vi "Begin.vi"(11 "Image Size":T1=enum."320x240") -> (0 "error out":errorcluster)   [LabVIEW 2012]
doc: "Called before other user functions, this VI is expected to open initial I/O refnums, load in file data, and do all program initialization. Notice that the <B>error out</B> terminal is simply used for data flow. Wiring it to other structures or subVIs ensures that this VI runs first."
uses:
  <vilib>/Rock Robotics/WPI/Camera/WPI_CameraImageSize.ctl
  <vilib>/Rock Robotics/WPI/DriverStation/WPI_DriverStationRobotMode2.ctl
  <vilib>/Rock Robotics/SystemInterfaces/DIO/FPGA_DIOPWMChannel.ctl
  <vilib>/Rock Robotics/WPI/Joystick/WPI_JoystickDeviceEnum.ctl
  <vilib>/Rock Robotics/WPI/Relay/WPI_RelayDirection.ctl
  <vilib>/Rock Robotics/SystemInterfaces/DIO/FPGA_DIORelayChannel.ctl
  <vilib>/Rock Robotics/SystemInterfaces/Typedef/FPGA_TypedefDigitalModule.ctl
  <vilib>/Rock Robotics/SystemInterfaces/AI/FPGA_AIChannel.ctl
  <vilib>/Rock Robotics/SystemInterfaces/AI/FPGA_AIGyroChannel.ctl
  <vilib>/Rock Robotics/SystemInterfaces/DIO/FPGA_DIOChannel.ctl
  Robot Global Data.vi
  <vilib>/Rock Robotics/WPI/MotorControl/WPI_MotorControlOpen Victor.vi
  <vilib>/Rock Robotics/WPI/Camera/WPI_CameraFrameRate.ctl
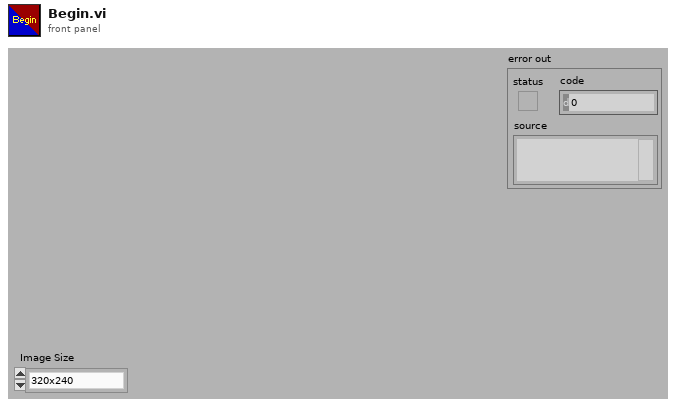
[diagram p1: front panel]
types:
  T1 = typedef "WPI_CameraImageSize.ctl" = enum16{"640x480", "320x240", "160x120"}
  T2 = typedef "FPGA_TypedefDigitalModule.ctl" = enum16{"Digital Module 1", "Digital Module 2"}
  T3 = typedef "FPGA_DIOPWMChannel.ctl" = enum8{"PWM 1", "PWM 2", "PWM 3", "PWM 4", "PWM 5", "PWM 6", "PWM 7", "PWM 8", "PWM 9", "PWM 10", "Invalid"}
  T4 = typedef "FPGA_DIORelayChannel.ctl" = enum8{"Relay 1", "Relay 2", "Relay 3", "Relay 4", "Relay 5", "Relay 6", "Relay 7", "Relay 8", "Invalid"}
  T5 = typedef "WPI_RelayDirection.ctl" = enum16{"Both directions", "Forward only", "Reverse only"}
  T6 = typedef "FPGA_DIOChannel.ctl" = enum8{"DIO 1", "DIO 2", "DIO 3", "DIO 4", "DIO 5", "DIO 6", "DIO 7", "DIO 8", "DIO 9", "DIO 10", "DIO 11", "DIO 12", "DIO 13", "DIO 14", "Invalid"}
  T7 = typedef "FPGA_AIChannel.ctl" = enum8{"AI 1", "AI 2", "AI 3", "AI 4", "AI 5", "AI 6", "AI 7", "AI 8", "Invalid"}
  T8 = typedef "FPGA_AIGyroChannel.ctl" = enum8{"AI 1", "AI 2", "Invalid"}
  T9 = typedef "WPI_JoystickDeviceEnum.ctl" = enum16{"USB 1", "USB 2", "USB 3", "USB 4", "Kinect 1", "Kinect 2"}
  T10 = typedef "WPI_DriverStationRobotMode2.ctl" = enum16{"Autonomous Disabled", "Autonomous Enabled", "Teleop Disabled", "Teleop Enabled", "Timeout", "Finish", "Test Disabled", "Test Enabled"}
  T11 = typedef "WPI_RelayDevRef.ctl" = cluster{"DevStatus":errorcluster, "Relay Channel":T4, "Digital Module":T2, "Relay Direction":T5}
  T12 = typedef "WPI_CameraFrameRate.ctl" = u32
  T13 = typedef "WPI_CameraDevRef.ctl" = cluster{"Camera Address":string, "CameraStatus":errorcluster, "Acquire Image Notifier":refnum<notifier>}
  T14 = typedef "WPI_MotorControlDeviceRef.ctl" = cluster{"DeviceStatus":errorcluster, "Type":enum16{"PWM", "CAN"}, "PWM":cluster{"Digital Module":T2, "PWM Channel":T3, "DeadBand":T15}, "CAN":cluster{"Device Number":u8, "Control Mode":T16, "Semaphore":T17, "Max Vout":dbl}, "Invert":bool, "TransformRef":T18, "InvTransformRef":T18}
  T15 = typedef "WPI_PWMDeadband.ctl" = cluster{"Name":string, "maxPositivePwm":i32, "minPositivePwm":i32, "centerPwm":i32, "maxNegativePwm":i32, "minNegativePwm":i32, "angularRange":u16}
  T16 = typedef "WPI_CANJaguar_ControlMode.ctl" = enum8{"Percent VBus", "Current", "Speed", "Position", "Voltage"}
  T17 = typedef "Semaphore RefNum" = refnum<k1>
  T18 = typedef "WPI_PWMTransform_ConPane.ctl" = refnum<vi>
  T19 = cluster{"Setpoint 1":dbl, "Setpoint 2":dbl, "Setpoint 3":dbl, "Setpoint 4":dbl, "RotLow":dbl, "RotHigh":dbl, "ExtLow":dbl, "ExtHigh":dbl}
  T20 = cluster{"FlipperLeftUp":dbl, "FlipperLeftDown":dbl, "FlipperRightUp":dbl, "FlipperRightDown":dbl, "KickerLeftBack":dbl, "KickerLeftForward":dbl, "KickerRightBack":dbl, "KickerRightForward":dbl}
  T21 = typedef "WPI_JoystickDevRef.ctl" = cluster{"Device":T9}
  T22 = typedef "WPI_ServoDeviceRef.ctl" = cluster{"DeviceStatus":errorcluster, "Digital Module":T2, "PWM Channel":T3, "DeadBand":T15}
  T23 = typedef "WPI_DigitalInputDevRef.ctl" = cluster{"DevStatus":errorcluster, "DIO Channel":T6, "Digital Module":T2}
  T24 = typedef "WPI_AnalogChannelDevRef.ctl" = cluster{"DevStatus":errorcluster, "Analog Module":T25, "Analog Channel":T7}
  T25 = typedef "FPGA_TypedefAnalogModule.ctl" = enum16{"Analog Module 1", "Analog Module 2"}
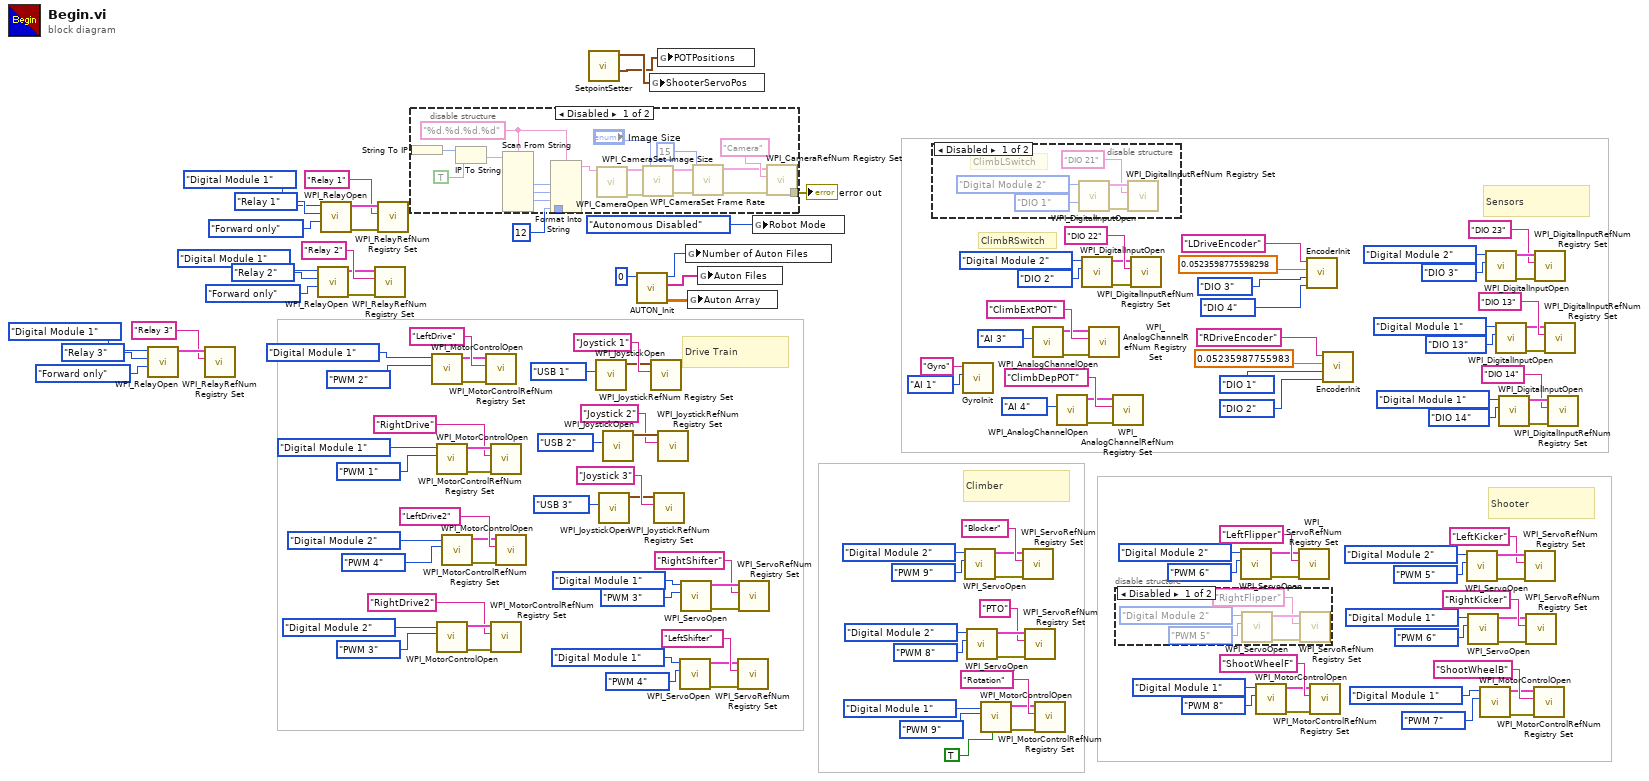
[diagram p0: block diagram]
diagram:
  # "ClimbRSwitch"
  # "Shooter"
  # "Drive Train"
  # "Climber"
  # "Sensors"
  n1 = call <vilib>:"WPI_RelayOpen.vi"("Relay Direction"=WPI_RelayDirection."Forward only", "Relay Channel"=FPGA_DIORelayChannel."Relay 3", "Digital Module (Module 1)"=FPGA_TypedefDigitalModule."Digital Module 1") -> ("RelayDevRef"=w14:T11)  [unwired: 7 in, 1 out]
  n2 = call <vilib>:"WPI_RelayRefNum Registry Set.vi"("refnum name"="Relay 3", "RelayDevRef"=w14) -> ()  [unwired: 8 in, 2 out]
  n3 = call <vilib>:"WPI_RelayOpen.vi"("Relay Direction"=WPI_RelayDirection."Forward only", "Relay Channel"=FPGA_DIORelayChannel."Relay 2", "Digital Module (Module 1)"=FPGA_TypedefDigitalModule."Digital Module 1") -> ("error out"=w106:errorcluster, "RelayDevRef"=w107:T11)  [unwired: 7 in]
  n4 = call <vilib>:"WPI_RelayOpen.vi"("Relay Direction"=WPI_RelayDirection."Forward only", "Relay Channel"=FPGA_DIORelayChannel."Relay 1", "Digital Module (Module 1)"=FPGA_TypedefDigitalModule."Digital Module 1") -> ("error out"=w64:errorcluster, "RelayDevRef"=w63:T11)  [unwired: 7 in]
  n5 = call <vilib>:"WPI_RelayRefNum Registry Set.vi"("error in (no error)"=w106, "refnum name"="Relay 2", "RelayDevRef"=w107) -> ()  [unwired: 7 in, 2 out]
  n6 = call <vilib>:"WPI_RelayRefNum Registry Set.vi"("error in (no error)"=w64, "refnum name"="Relay 1", "RelayDevRef"=w63) -> ()  [unwired: 7 in, 2 out]
  n7 = disable-structure shown="Disabled" {
    disable-tunnel: 12 ("Compression") -> [w155 _]
    disable-tunnel: [w145 _] -> w65
    frame Disabled {
      w154 = "%d.%d.%d.%d" ("format string")
      n8 = String To IP() -> (0:w161:u32)  [unwired: 1 in]
      n9 = IP To String(1:TRUE ("dot notation? (F)"), 2:w161) -> (0:w159:string)
      n10 = Scan From String(format string=w154, input string=w159) -> (output 1=w158:i32, output 2=w157:i32, output 3=w156:i32)  [unwired: 7 in, 3 out]
      n11 = Format Into String(format string=w154, w158, w157, w156, w155) -> (resulting string=w153:string)  [unwired: 2 in, 1 out]
      n12 = call <vilib>:"WPI_CameraOpen.vi"("Camera Address"=w153) -> ("error out"=w152:errorcluster, "CameraDevRef"=w151:T13)  [unwired: 1 in, 8 out]
      n13 = call <vilib>:"WPI_CameraSet Image Size.vi"("error in (no error)"=w152, "Image Size"="Image Size", "CameraDevRef"=w151) -> ("error out"=w149:errorcluster, "CameraDevRef Out"=w150:T13)  [unwired: 7 out]
      n14 = call <vilib>:"WPI_CameraSet Frame Rate.vi"("error in (no error)"=w149, "Frame Rate (fps)"=T12 15, "CameraDevRef"=w150) -> ("error out"=w148:errorcluster, "CameraDevRef Out"=w147:T13)  [unwired: 7 out]
      n15 = call <vilib>:"WPI_CameraRefNum Registry Set.vi"("error in (no error)"=w148, "refnum name"="Camera", "CameraDevRef"=w147) -> ("error out"=w145:errorcluster)  [unwired: 8 out]
    }
    frame Enabled {
    }
  }
  "error out" <- w65
  n16 = call-poly <vilib>:"WPI_MotorControlOpen.vi"("PWM Channel"=FPGA_DIOPWMChannel."PWM 2", "Digital Module (Module 1)"=FPGA_TypedefDigitalModule."Digital Module 1") -> ("error out"=w132:errorcluster, "MotorControlDeviceRef"=w133:T14)  [unwired: 8 in]
  n17 = call-poly <vilib>:"WPI_MotorControlOpen.vi"("PWM Channel"=FPGA_DIOPWMChannel."PWM 1", "Digital Module (Module 1)"=FPGA_TypedefDigitalModule."Digital Module 1") -> ("error out"=w139:errorcluster, "MotorControlDeviceRef"=w138:T14)  [unwired: 8 in]
  n18 = call-poly <vilib>:"WPI_MotorControlOpen.vi"("PWM Channel"=FPGA_DIOPWMChannel."PWM 3", "Digital Module (Module 1)"=FPGA_TypedefDigitalModule."Digital Module 2") -> ("error out"=w121:errorcluster, "MotorControlDeviceRef"=w120:T14)  [unwired: 8 in]
  n19 = call-poly <vilib>:"WPI_MotorControlOpen.vi"("PWM Channel"=FPGA_DIOPWMChannel."PWM 4", "Digital Module (Module 1)"=FPGA_TypedefDigitalModule."Digital Module 2") -> ("error out"=w112:errorcluster, "MotorControlDeviceRef"=w113:T14)  [unwired: 8 in]
  n20 = call <vilib>:"WPI_MotorControlRefNum Registry Set.vi"("error in (no error)"=w132, "refnum name"="LeftDrive", "MotorControlDevRef"=w133) -> ()  [unwired: 7 in, 2 out]
  n21 = call <vilib>:"WPI_MotorControlRefNum Registry Set.vi"("error in (no error)"=w139, "refnum name"="RightDrive", "MotorControlDevRef"=w138) -> ()  [unwired: 7 in, 2 out]
  n22 = call <vilib>:"WPI_MotorControlRefNum Registry Set.vi"("error in (no error)"=w121, "refnum name"="RightDrive2", "MotorControlDevRef"=w120) -> ()  [unwired: 7 in, 2 out]
  n23 = call <vilib>:"WPI_MotorControlRefNum Registry Set.vi"("error in (no error)"=w112, "refnum name"="LeftDrive2", "MotorControlDevRef"=w113) -> ()  [unwired: 7 in, 2 out]
  n24 = call "SetpointSetter.vi"() -> ("Arm Pos"=w1:T19, "Shooter Servo Pos"=w2:T20)  [unwired: 10 in]
  n25 = call <vilib>:"WPI_JoystickOpen.vi"("JoystickDevice"=WPI_JoystickDeviceEnum."USB 1") -> ("JoystickDevRef"=w123:T21)  [unwired: 10 in]
  n26 = call <vilib>:"WPI_JoystickOpen.vi"("JoystickDevice"=WPI_JoystickDeviceEnum."USB 3") -> ("JoystickDevRef"=w129:T21)  [unwired: 10 in]
  n27 = call <vilib>:"WPI_JoystickOpen.vi"("JoystickDevice"=WPI_JoystickDeviceEnum."USB 2") -> ("JoystickDevRef"=w128:T21)  [unwired: 10 in]
  n28 = call "AUTON_Init.vi"("Default File"=0) -> ("Auton Array"=w140:dbl[][], "Auton Files"=w141:string[], "Number of Auton Files"=w142:i64)  [unwired: 8 in]
  n29 = global write "Robot Global Data.vi" "ShooterServoPos"(w2) -> ()
  n30 = call <vilib>:"WPI_JoystickRefNum Registry Set.vi"("refnum name"="Joystick 1", "JoystickDevRef"=w123) -> ()  [unwired: 8 in, 2 out]
  n31 = call <vilib>:"WPI_JoystickRefNum Registry Set.vi"("refnum name"="Joystick 3", "JoystickDevRef"=w129) -> ()  [unwired: 8 in, 2 out]
  n32 = global write "Robot Global Data.vi" "POTPositions"(w1) -> ()
  n33 = call <vilib>:"WPI_JoystickRefNum Registry Set.vi"("refnum name"="Joystick 2", "JoystickDevRef"=w128) -> ()  [unwired: 8 in, 2 out]
  n34 = call <vilib>:"WPI_ServoOpen.vi"("PWM Channel"=FPGA_DIOPWMChannel."PWM 4", "Digital Module (Module 1)"=FPGA_TypedefDigitalModule."Digital Module 1") -> ("error out"=w105:errorcluster, "ServoDeviceRef"=w98:T22)  [unwired: 8 in]
  n35 = call <vilib>:"WPI_ServoOpen.vi"("PWM Channel"=FPGA_DIOPWMChannel."PWM 3", "Digital Module (Module 1)"=FPGA_TypedefDigitalModule."Digital Module 1") -> ("error out"=w104:errorcluster, "ServoDeviceRef"=w103:T22)  [unwired: 8 in]
  n36 = global write "Robot Global Data.vi" "Number of Auton Files"(w142) -> ()
  n37 = global write "Robot Global Data.vi" "Auton Array"(w140) -> ()
  n38 = global write "Robot Global Data.vi" "Auton Files"(w141) -> ()
  n39 = call <vilib>:"WPI_ServoRefNum Registry Set.vi"("error in (no error)"=w105, "refnum name"="LeftShifter", "ServoDeviceRef"=w98) -> ()  [unwired: 7 in, 2 out]
  n40 = call <vilib>:"WPI_ServoRefNum Registry Set.vi"("error in (no error)"=w104, "refnum name"="RightShifter", "ServoDeviceRef"=w103) -> ()  [unwired: 7 in, 2 out]
  n41 = global write "Robot Global Data.vi" "Robot Mode"(WPI_DriverStationRobotMode2."Autonomous Disabled" ("Robot Mode")) -> ()
  n42 = disable-structure shown="Disabled" {
    frame Disabled {
      # "ClimbLSwitch"
      n43 = call <vilib>:"WPI_DigitalInputOpen.vi"("DIO Channel"=FPGA_DIOChannel."DIO 1", "Digital Module (Module 1)"=FPGA_TypedefDigitalModule."Digital Module 2") -> ("error out"=w165:errorcluster, "DigitalInputDevRef"=w166:T23)  [unwired: 8 in]
      n44 = call <vilib>:"WPI_DigitalInputRefNum Registry Set.vi"("error in (no error)"=w165, "refnum name"="DIO 21", "DigitalInputDevRef"=w166) -> ()  [unwired: 7 in, 2 out]
    }
    frame Enabled {
    }
  }
  n45 = call "GyroInit.vi"("refnum name"="Gyro", "Analog Channel"=FPGA_AIGyroChannel."AI 1") -> ()  [unwired: 8 in]
  n46 = call <vilib>:"WPI_ServoOpen.vi"("PWM Channel"=FPGA_DIOPWMChannel."PWM 9", "Digital Module (Module 1)"=FPGA_TypedefDigitalModule."Digital Module 2") -> ("error out"=w4:errorcluster, "ServoDeviceRef"=w5:T22)  [unwired: 8 in]
  n47 = call <vilib>:"WPI_ServoOpen.vi"("PWM Channel"=FPGA_DIOPWMChannel."PWM 8", "Digital Module (Module 1)"=FPGA_TypedefDigitalModule."Digital Module 2") -> ("error out"=w83:errorcluster, "ServoDeviceRef"=w82:T22)  [unwired: 8 in]
  n48 = call-poly <vilib>:"WPI_MotorControlOpen.vi"("Invert"=TRUE, "PWM Channel"=FPGA_DIOPWMChannel."PWM 9", "Digital Module (Module 1)"=FPGA_TypedefDigitalModule."Digital Module 1") -> ("error out"=w88:errorcluster, "MotorControlDeviceRef"=w87:T14)  [unwired: 7 in]
  n49 = call <vilib>:"WPI_ServoRefNum Registry Set.vi"("error in (no error)"=w4, "refnum name"="Blocker", "ServoDeviceRef"=w5) -> ()  [unwired: 7 in, 2 out]
  n50 = call <vilib>:"WPI_ServoRefNum Registry Set.vi"("error in (no error)"=w83, "refnum name"="PTO", "ServoDeviceRef"=w82) -> ()  [unwired: 7 in, 2 out]
  n51 = call <vilib>:"WPI_AnalogChannelOpen.vi"("Analog Channel"=FPGA_AIChannel."AI 3") -> ("error out"=w67:errorcluster, "AIDeviceRef"=w68:T24)  [unwired: 9 in]
  n52 = call <vilib>:"WPI_MotorControlRefNum Registry Set.vi"("error in (no error)"=w88, "refnum name"="Rotation", "MotorControlDevRef"=w87) -> ()  [unwired: 7 in, 2 out]
  n53 = call <vilib>:"WPI_AnalogChannelOpen.vi"("Analog Channel"=FPGA_AIChannel."AI 4") -> ("error out"=w92:errorcluster, "AIDeviceRef"=w93:T24)  [unwired: 9 in]
  n54 = call <vilib>:"WPI_DigitalInputOpen.vi"("DIO Channel"=FPGA_DIOChannel."DIO 2", "Digital Module (Module 1)"=FPGA_TypedefDigitalModule."Digital Module 2") -> ("error out"=w18:errorcluster, "DigitalInputDevRef"=w17:T23)  [unwired: 8 in]
  n55 = call <vilib>:"WPI_AnalogChannelRefNum Registry Set.vi"("error in (no error)"=w67, "refnum name"="ClimbExtPOT", "AIDeviceRef"=w68) -> ()  [unwired: 7 in, 2 out]
  n56 = call <vilib>:"WPI_AnalogChannelRefNum Registry Set.vi"("error in (no error)"=w92, "refnum name"="ClimbDepPOT", "AIDeviceRef"=w93) -> ()  [unwired: 7 in, 2 out]
  n57 = disable-structure shown="Disabled" {
    frame Disabled {
      n58 = call <vilib>:"WPI_ServoOpen.vi"("PWM Channel"=FPGA_DIOPWMChannel."PWM 5", "Digital Module (Module 1)"=FPGA_TypedefDigitalModule."Digital Module 2") -> ("error out"=w173:errorcluster, "ServoDeviceRef"=w172:T22)  [unwired: 8 in]
      n59 = call <vilib>:"WPI_ServoRefNum Registry Set.vi"("error in (no error)"=w173, "refnum name"="RightFlipper", "ServoDeviceRef"=w172) -> ()  [unwired: 7 in, 2 out]
    }
    frame Enabled {
    }
  }
  n60 = call <vilib>:"WPI_DigitalInputRefNum Registry Set.vi"("error in (no error)"=w18, "refnum name"="DIO 22", "DigitalInputDevRef"=w17) -> ()  [unwired: 7 in, 2 out]
  n61 = call <vilib>:"WPI_ServoOpen.vi"("PWM Channel"=FPGA_DIOPWMChannel."PWM 6", "Digital Module (Module 1)"=FPGA_TypedefDigitalModule."Digital Module 2") -> ("error out"=w45:errorcluster, "ServoDeviceRef"=w46:T22)  [unwired: 8 in]
  n62 = call-poly <vilib>:"WPI_MotorControlOpen.vi"("PWM Channel"=FPGA_DIOPWMChannel."PWM 8", "Digital Module (Module 1)"=FPGA_TypedefDigitalModule."Digital Module 1") -> ("error out"=w56:errorcluster, "MotorControlDeviceRef"=w57:T14)  [unwired: 8 in]
  n63 = call <vilib>:"WPI_ServoRefNum Registry Set.vi"("error in (no error)"=w45, "refnum name"="LeftFlipper", "ServoDeviceRef"=w46) -> ()  [unwired: 7 in, 2 out]
  n64 = call "EncoderInit.vi"("refnum name"="LDriveEncoder", "DistancePerCount"=0.0523598775598298, "DIO Channel"=FPGA_DIOChannel."DIO 3", "DIO Channel 2"=FPGA_DIOChannel."DIO 4") -> ()  [unwired: 7 in]
  n65 = call <vilib>:"WPI_MotorControlRefNum Registry Set.vi"("error in (no error)"=w56, "refnum name"="ShootWheelF", "MotorControlDevRef"=w57) -> ()  [unwired: 7 in, 2 out]
  n66 = call "EncoderInit.vi"("refnum name"="RDriveEncoder", "DistancePerCount"=0.05235987755983, "DIO Channel"=FPGA_DIOChannel."DIO 1", "DIO Channel 2"=FPGA_DIOChannel."DIO 2") -> ()  [unwired: 7 in]
  n67 = call <vilib>:"WPI_ServoOpen.vi"("PWM Channel"=FPGA_DIOPWMChannel."PWM 5", "Digital Module (Module 1)"=FPGA_TypedefDigitalModule."Digital Module 2") -> ("error out"=w40:errorcluster, "ServoDeviceRef"=w39:T22)  [unwired: 8 in]
  n68 = call <vilib>:"WPI_ServoOpen.vi"("PWM Channel"=FPGA_DIOPWMChannel."PWM 6", "Digital Module (Module 1)"=FPGA_TypedefDigitalModule."Digital Module 1") -> ("error out"=w35:errorcluster, "ServoDeviceRef"=w41:T22)  [unwired: 8 in]
  n69 = call-poly <vilib>:"WPI_MotorControlOpen.vi"("PWM Channel"=FPGA_DIOPWMChannel."PWM 7", "Digital Module (Module 1)"=FPGA_TypedefDigitalModule."Digital Module 1") -> ("error out"=w52:errorcluster, "MotorControlDeviceRef"=w51:T14)  [unwired: 8 in]
  n70 = call <vilib>:"WPI_DigitalInputOpen.vi"("DIO Channel"=FPGA_DIOChannel."DIO 3", "Digital Module (Module 1)"=FPGA_TypedefDigitalModule."Digital Module 2") -> ("error out"=w20:errorcluster, "DigitalInputDevRef"=w23:T23)  [unwired: 8 in]
  n71 = call <vilib>:"WPI_DigitalInputOpen.vi"("DIO Channel"=FPGA_DIOChannel."DIO 13", "Digital Module (Module 1)"=FPGA_TypedefDigitalModule."Digital Module 1") -> ("error out"=w33:errorcluster, "DigitalInputDevRef"=w32:T23)  [unwired: 8 in]
  n72 = call <vilib>:"WPI_DigitalInputOpen.vi"("DIO Channel"=FPGA_DIOChannel."DIO 14", "Digital Module (Module 1)"=FPGA_TypedefDigitalModule."Digital Module 1") -> ("error out"=w26:errorcluster, "DigitalInputDevRef"=w27:T23)  [unwired: 8 in]
  n73 = call <vilib>:"WPI_ServoRefNum Registry Set.vi"("error in (no error)"=w40, "refnum name"="LeftKicker", "ServoDeviceRef"=w39) -> ()  [unwired: 7 in, 2 out]
  n74 = call <vilib>:"WPI_ServoRefNum Registry Set.vi"("error in (no error)"=w35, "refnum name"="RightKicker", "ServoDeviceRef"=w41) -> ()  [unwired: 7 in, 2 out]
  n75 = call <vilib>:"WPI_MotorControlRefNum Registry Set.vi"("error in (no error)"=w52, "refnum name"="ShootWheelB", "MotorControlDevRef"=w51) -> ()  [unwired: 7 in, 2 out]
  n76 = call <vilib>:"WPI_DigitalInputRefNum Registry Set.vi"("error in (no error)"=w20, "refnum name"="DIO 23", "DigitalInputDevRef"=w23) -> ()  [unwired: 7 in, 2 out]
  n77 = call <vilib>:"WPI_DigitalInputRefNum Registry Set.vi"("error in (no error)"=w33, "refnum name"="DIO 13", "DigitalInputDevRef"=w32) -> ()  [unwired: 7 in, 2 out]
  n78 = call <vilib>:"WPI_DigitalInputRefNum Registry Set.vi"("error in (no error)"=w26, "refnum name"="DIO 14", "DigitalInputDevRef"=w27) -> ()  [unwired: 7 in, 2 out]
